vi "InRangeOfTarget.vi"(1 "Tolerance":dbl, 2 "Target":dbl, 3 "Value":dbl) -> (0 "Is In Range":bool)   [LabVIEW 2016]
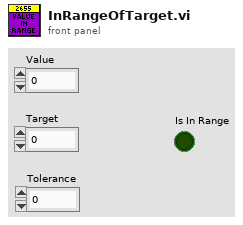
[diagram p1: front panel]
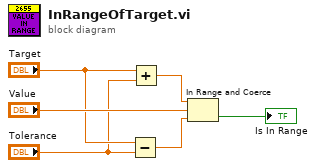
[diagram p0: block diagram]
diagram:
  n1 = Subtract(x="Target", y="Tolerance") -> (x-y=w4:dbl)
  n2 = Add(x="Target", y="Tolerance") -> (x+y=w5:dbl)
  n3 = In Range and Coerce(upper limit=w5, x="Value", lower limit=w4) -> (In Range?=→"Is In Range":bool)  [unwired: 1 out]
